vi "StreamDAQ.vi"(0 "Stream Data Type":dbl[][](array[numeric]), 1 "Control refDes array":string[][](array[string]), 5 "control data type":variant, 7 "Logging Queue":refnum<queue>, 9 "StreamTypeDef":T1, 11 "error in":errorcluster) -> (4 "control data out":variant, 10 "StreamTypeDef":T1, 15 "error out":errorcluster)   [LabVIEW 2024]
uses:
  Control/StreamTypeDef.ctl
  Control/streamIO_states.ctl
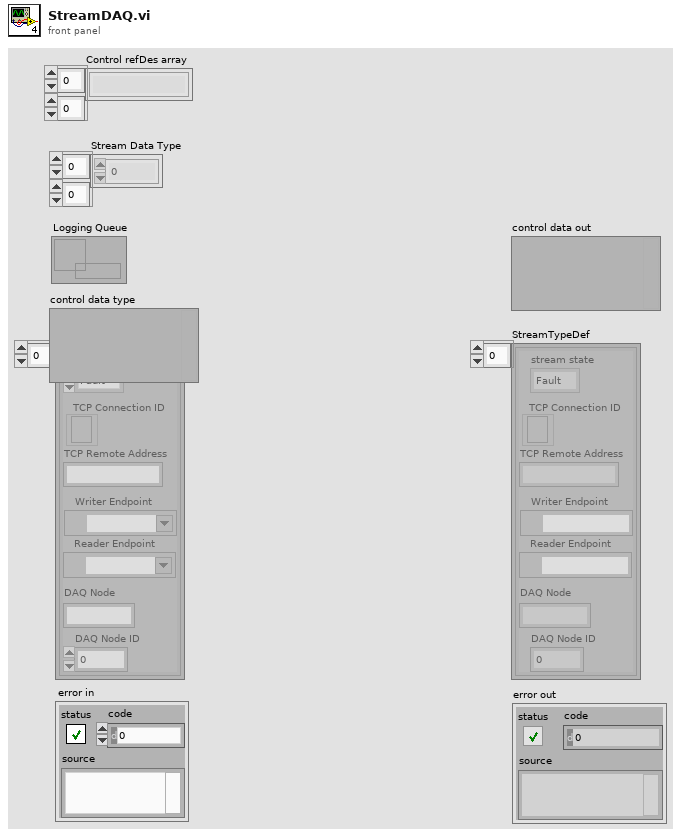
[diagram p1: front panel]
types:
  T1 = typedef "StreamTypeDef.ctl" = cluster{"stream state":T2, "TCP Remote Address":string, "TCP Connection ID":refnum<k5>, "Reader Endpoint":refnum<k21>, "Writer Endpoint":refnum<k21>, "DAQ Node":string, "DAQ Node ID":i32}[]
  T2 = typedef "streamIO_states.ctl" = enum16{"Fault", "Initilize", "Stream", "Close"}
  T3 = cluster{"stream state":T2, "TCP Remote Address":string, "TCP Connection ID":refnum<k5>, "Reader Endpoint":refnum<k21>, "Writer Endpoint":refnum<k21>, "DAQ Node":string, "DAQ Node ID":i32}
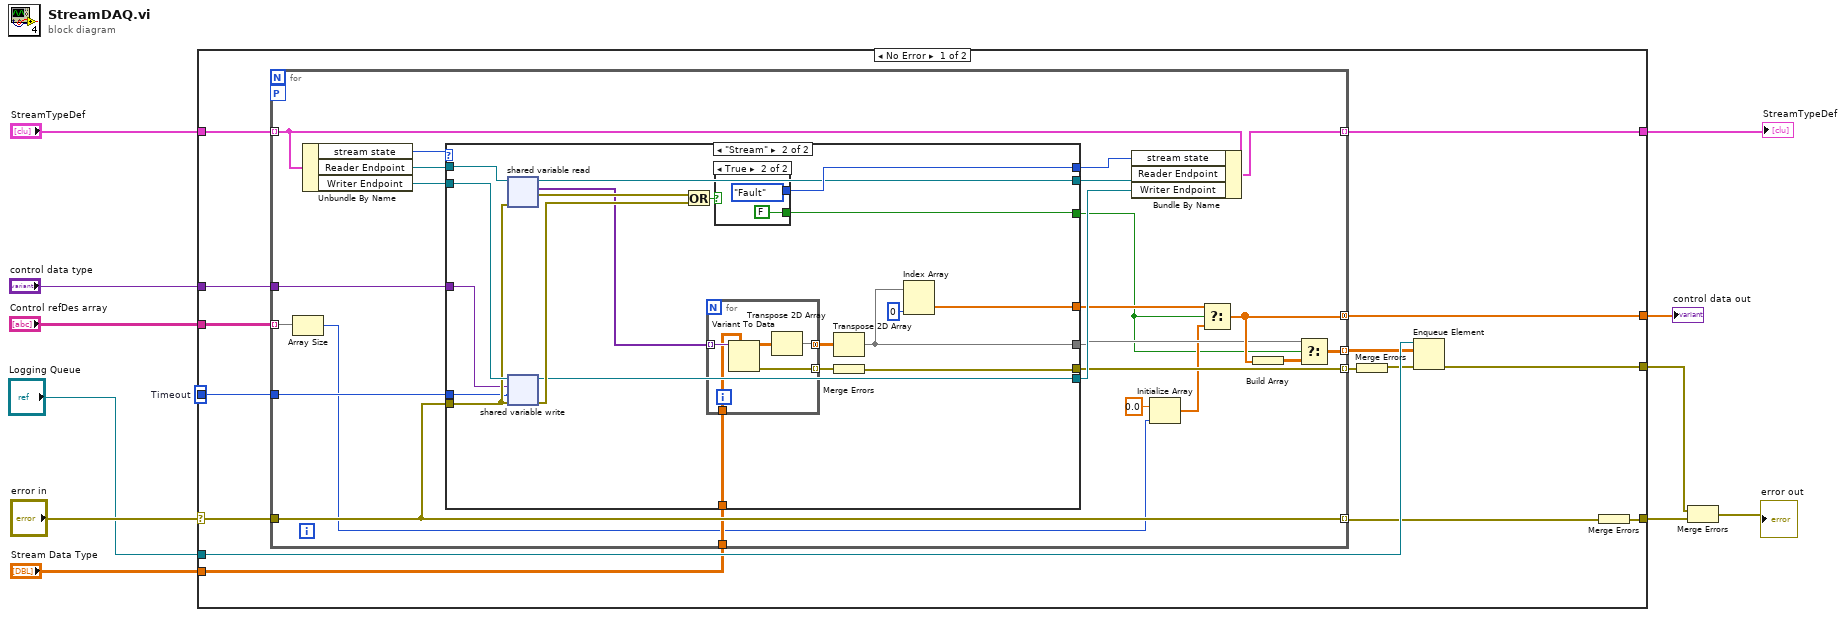
[diagram p0: block diagram]
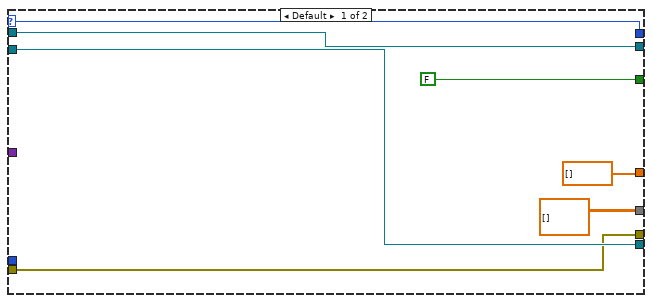
[diagram p2: hidden frame]
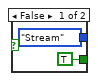
[diagram p3: hidden frame]
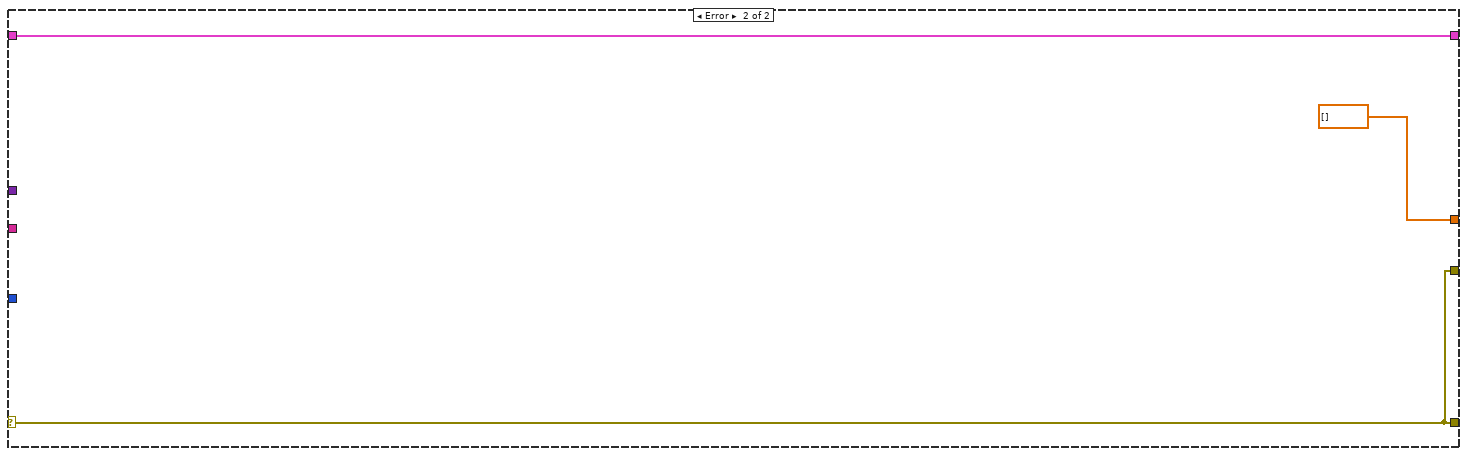
[diagram p4: hidden frame]
diagram:
  w7 = 2  # Timeout
  n1 = case shown="No Error" "error in" {
    selector: "error in" -> [w24 w89]
    tunnel: "StreamTypeDef" -> [w13 w88]
    tunnel: [w27 w88] -> w11
    tunnel: [w18 w89] -> w10
    tunnel: "control data type" -> [w26 _]
    tunnel: w7 -> [w25 _]
    tunnel: "Logging Queue" -> [w23 _]
    tunnel: "Stream Data Type" -> [w22 _]
    tunnel: [w19 w89] -> w3
    tunnel: [w15 dbl[] []] -> w2
    tunnel: "Control refDes array" -> [w14 _]
    frame No Error {
      n2 = for {
        tunnel: w13 -> [w45] mode=indexing
        tunnel: [w44] -> w27 mode=indexing
        tunnel: [w47] -> w17 mode=indexing
        tunnel: w24 -> [w47]
        tunnel: w26 -> [w46]
        tunnel: w25 -> [w40]
        tunnel: w22 -> [w39]
        tunnel: [w34] -> w16 mode=indexing
        tunnel: [w38] -> w20 mode=indexing
        tunnel: [w32] -> w15 mode=concatenating
        tunnel: w14 -> [w37] mode=indexing
        workers-P: _ -> [_]
        n3 = Array Size(array=w37) -> (size(s)=w36:i32)
        n4 = Unbundle By Name(w45) -> ("stream state"=w50:T2, "Reader Endpoint"=w49:refnum<k21>, "Writer Endpoint"=w48:refnum<k21>)
        n5 = case shown="\"Stream\"" w50 {
          selector: w50 -> [w55 _]
          tunnel: w49 -> [w57 w77]
          tunnel: w48 -> [w56 w76]
          tunnel: w47 -> [w54 w75]
          tunnel: w46 -> [_ w74]
          tunnel: [w55 w70] -> w43
          tunnel: [w57 w69] -> w42
          tunnel: [w56 w68] -> w41
          tunnel: w40 -> [_ w67]
          tunnel: w39 -> [_ w65]
          tunnel: [dbl[][] [] w60] -> w30
          tunnel: [w54 w63] -> w38
          tunnel: [dbl[] [] w59] -> w31
          tunnel: [FALSE w58] -> w28
          frame Default {
          }
          frame "Stream" {
            n6 = shared-variable-read(w77, w75) -> (w69:refnum<k21>, w72:errorcluster, w66:variant[])  [unwired: 2 in, 1 out]
            n7 = shared-variable-write(w76, w75, w74, w67) -> (w68:refnum<k21>, w71:errorcluster)  [unwired: 1 out]
            n8 = Or(x=w72, y=w71) -> (x .or. y?=w73:bool)
            n9 = for {
              tunnel: w66 -> [w82] mode=indexing
              tunnel: w65 -> [w81]
              tunnel: [w79] -> w64 mode=concatenating
              tunnel: [w78] -> w62 mode=indexing
              n10 = Variant To Data(type=w81, Variant=w82) -> (data=w80:dbl[][], error out=w78:errorcluster)  [unwired: 1 in]
              n11 = Transpose 2D Array(2D array=w80) -> (transposed array=w79:dbl[][])
            }
            n12 = case shown="True" w73 {
              tunnel: [streamIO_states."Stream" ("stream state") streamIO_states."Fault" ("stream state")] -> w70
              tunnel: [TRUE FALSE] -> w58
              frame False {
              }
              frame True {
              }
            }
            n13 = Transpose 2D Array(2D array=w64) -> (transposed array=w60:dbl[][])
            n14 = Merge Errors(w62) -> (w63:errorcluster)
            n15 = Index Array(array=w60, index (col)=0) -> (element=w59:dbl[])  [unwired: 1 in]
          }
        }
        n16 = Bundle By Name(cluster=w45, "stream state"=w43, "Reader Endpoint"=w42, "Writer Endpoint"=w41) -> (w44:T3)
        n17 = Initialize Array(0.0 ("element"), w36) -> (w29:dbl[])
        n18 = Select(t=w31, s=w28, f=w29) -> (s? t:f=w32:dbl[])
        n19 = Build Array(w32) -> (w33:dbl[][])
        n20 = Select(t=w30, s=w28, f=w33) -> (s? t:f=w34:dbl[][])
      }
      n21 = Merge Errors(w20) -> (w21:errorcluster)
      n22 = Enqueue Element(queue=w23, element=w16, error in (no error)=w21) -> (error out=w19:errorcluster)  [unwired: 1 in, 2 out]
      n23 = Merge Errors(w17) -> (w18:errorcluster)
    }
    frame Error {
    }
  }
  "StreamTypeDef" <- w11
  "control data out" <- w2
  n24 = Merge Errors(w3, w10) -> (→"error out":errorcluster)
